vi "parcour_erstellen.vi"() -> (1 "XY_Parcout":cluster{"x":dbl[], "y":dbl[]}[](array[cluster]), 3 "parcour_Liste out":refnum<class "parcour_Liste.lvclass">)   [LabVIEW 2019]
uses:
  parcour_liste/parcour_Liste.lvclass
  Kreisquadrant/Kreisquadrant.lvclass
  C:/Users/juerg.keller1/Documents/FHNW/STUDPROJ/2020-2021/MTB/labview/simulation/parcour/Parcour_element.lvclass
  Gerade/Gerade.lvclass
  mode_Q.ctl
  parcour/Parcour_element.lvclass
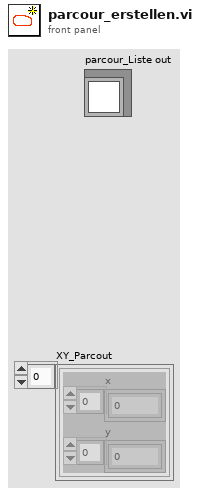
[diagram p1: front panel]
types:
  T1 = typedef "mode_Q.ctl" = enum16{"init", "get"}
  T2 = enum16{"oben_rechts", "oben_links", "unten_links", "unten_rechts"}
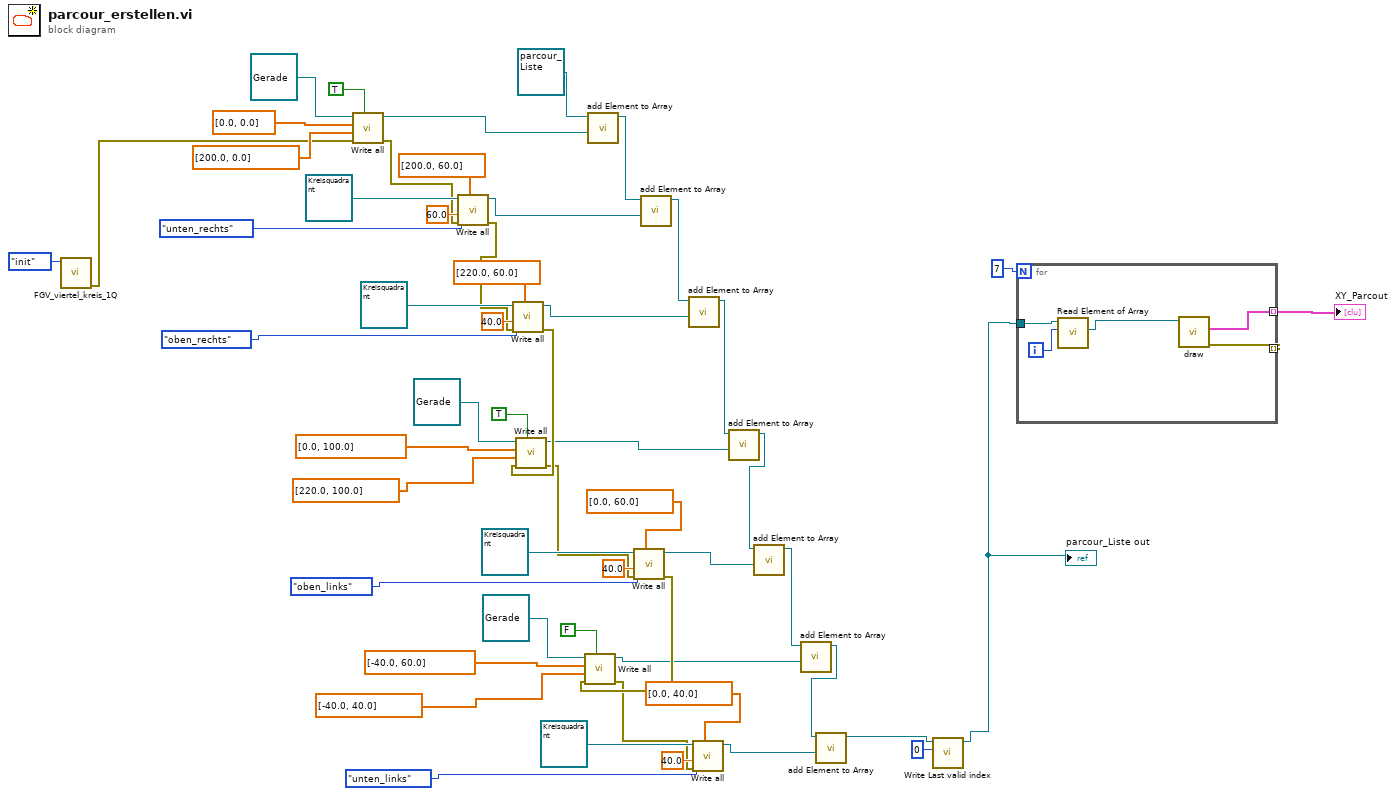
[diagram p0: block diagram]
diagram:
  n1 = call "FGV_viertel_kreis_1Q.vi"("mode"=mode_Q."init") -> ("error out"=w26:errorcluster)  [unwired: 8 in, 2 out]
  n2 = call-dynamic "Write all.vi"("horizontal"=TRUE, "error in (no error)"=w26, "Endpunkt"=dbl[] [200.0, 0.0] ("Startpunkt"), "Startpunkt"=dbl[] [0.0, 0.0], "Gerade in"=refnum<class "Gerade.lvclass"> refnum) -> ("error out"=w25:errorcluster, "Gerade out"=w20:refnum<class "Gerade.lvclass">)  [unwired: 5 in]
  n3 = call-dynamic "Write all.vi"("Zentrum"=dbl[] [200.0, 60.0], "error in (no error)"=w25, "Radius"=60.0, "Sektor"=T2."unten_rechts", "Kreisquadrant in"=refnum<class "Kreisquadrant.lvclass"> refnum) -> ("error out"=w24:errorcluster, "Kreisquadrant out"=w8:refnum<class "Kreisquadrant.lvclass">)  [unwired: 5 in]
  n4 = call-dynamic "Write all.vi"("Zentrum"=dbl[] [220.0, 60.0], "error in (no error)"=w24, "Radius"=40.0, "Sektor"=T2."oben_rechts", "Kreisquadrant in"=refnum<class "Kreisquadrant.lvclass"> refnum) -> ("error out"=w23:errorcluster, "Kreisquadrant out"=w9:refnum<class "Kreisquadrant.lvclass">)  [unwired: 5 in]
  n5 = call-dynamic "Write all.vi"("horizontal"=TRUE, "error in (no error)"=w23, "Endpunkt"=dbl[] [220.0, 100.0] ("Startpunkt"), "Startpunkt"=dbl[] [0.0, 100.0], "Gerade in"=refnum<class "Gerade.lvclass"> refnum) -> ("error out"=w22:errorcluster, "Gerade out"=w10:refnum<class "Gerade.lvclass">)  [unwired: 5 in]
  n6 = call-dynamic "add Element to Array.vi"("Parcour_element.lvclass"=w20, "parcour_Liste in"=refnum<class "parcour_Liste.lvclass"> refnum) -> ("parcour_Liste out"=w17:refnum<class "parcour_Liste.lvclass">)  [unwired: 8 in, 1 out]
  n7 = call-dynamic "Write all.vi"("Zentrum"=dbl[] [0.0, 60.0], "error in (no error)"=w22, "Radius"=40.0, "Sektor"=T2."oben_links", "Kreisquadrant in"=refnum<class "Kreisquadrant.lvclass"> refnum) -> ("error out"=w19:errorcluster, "Kreisquadrant out"=w6:refnum<class "Kreisquadrant.lvclass">)  [unwired: 5 in]
  n8 = call-dynamic "Write all.vi"("horizontal"=FALSE, "error in (no error)"=w19, "Endpunkt"=dbl[] [-40.0, 40.0] ("Startpunkt"), "Startpunkt"=dbl[] [-40.0, 60.0], "Gerade in"=refnum<class "Gerade.lvclass"> refnum) -> ("error out"=w18:errorcluster, "Gerade out"=w5:refnum<class "Gerade.lvclass">)  [unwired: 5 in]
  n9 = call-dynamic "add Element to Array.vi"("Parcour_element.lvclass"=w8, "parcour_Liste in"=w17) -> ("parcour_Liste out"=w16:refnum<class "parcour_Liste.lvclass">)  [unwired: 8 in, 1 out]
  n10 = call-dynamic "add Element to Array.vi"("Parcour_element.lvclass"=w9, "parcour_Liste in"=w16) -> ("parcour_Liste out"=w15:refnum<class "parcour_Liste.lvclass">)  [unwired: 8 in, 1 out]
  n11 = call-dynamic "Write all.vi"("Zentrum"=dbl[] [0.0, 40.0], "error in (no error)"=w18, "Radius"=40.0, "Sektor"=T2."unten_links", "Kreisquadrant in"=refnum<class "Kreisquadrant.lvclass"> refnum) -> ("Kreisquadrant out"=w11:refnum<class "Kreisquadrant.lvclass">)  [unwired: 5 in, 1 out]
  n12 = call-dynamic "add Element to Array.vi"("Parcour_element.lvclass"=w10, "parcour_Liste in"=w15) -> ("parcour_Liste out"=w14:refnum<class "parcour_Liste.lvclass">)  [unwired: 8 in, 1 out]
  n13 = call-dynamic "add Element to Array.vi"("Parcour_element.lvclass"=w6, "parcour_Liste in"=w14) -> ("parcour_Liste out"=w13:refnum<class "parcour_Liste.lvclass">)  [unwired: 8 in, 1 out]
  n14 = call-dynamic "add Element to Array.vi"("Parcour_element.lvclass"=w5, "parcour_Liste in"=w13) -> ("parcour_Liste out"=w12:refnum<class "parcour_Liste.lvclass">)  [unwired: 8 in, 1 out]
  n15 = call-dynamic "add Element to Array.vi"("Parcour_element.lvclass"=w11, "parcour_Liste in"=w12) -> ("parcour_Liste out"=w4:refnum<class "parcour_Liste.lvclass">)  [unwired: 8 in, 1 out]
  n16 = call-dynamic "Write Last valid index.vi"("Last valid index"=0, "parcour_Liste in"=w4) -> ("parcour_Liste out"=w1:refnum<class "parcour_Liste.lvclass">)  [unwired: 8 in, 1 out]
  "parcour_Liste out" <- w1
  n17 = for {
    N: 7 -> [_]
    tunnel: [w60] -> _ mode=indexing
    tunnel: [w59] -> w2 mode=indexing
    tunnel: w1 -> [w58]
    i -> [w57]
    n18 = call-dynamic "Read Element of Array.vi"("index"=w57, "parcour_Liste in"=w58) -> ("Parcour_element.lvclass"=w56:refnum<class "Parcour_element.lvclass">)  [unwired: 7 in, 2 out]
    n19 = call-dynamic "draw.vi"("Parcour_element in"=w56) -> ("error out"=w60:errorcluster, "element"=w59:cluster{"x":dbl[], "y":dbl[]})  [unwired: 8 in, 1 out]
  }
  "XY_Parcout" <- w2
